vi "get_id.vi"(11 "node":refnum<class "Node.lvclass">) -> (1 "label":string, 2 "node-id":refnum<class "ID.lvclass">)   [LabVIEW 2020, in "graph.lvlib" / "Node.lvclass"]
uses:
  Node.lvclass
  ID/ID.lvclass
  Node.lvclass/Node.ctl
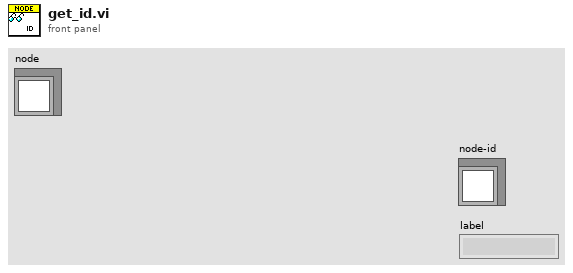
[diagram p1: front panel]
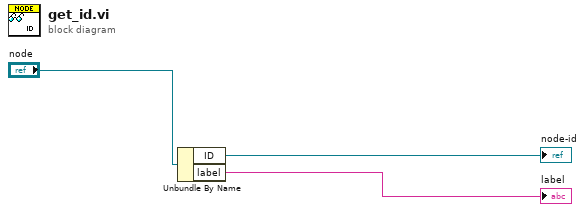
[diagram p0: block diagram]
diagram:
  n1 = Unbundle By Name("node") -> ("ID"=→"node-id":refnum<class "ID.lvclass">, "label"=→"label":string)
